vi "Ports Submenu.vi"(11 "menu reference":refnum<k9>) -> ()   [LabVIEW 2017]
panel:
  in  "error in (no error)":errorcluster
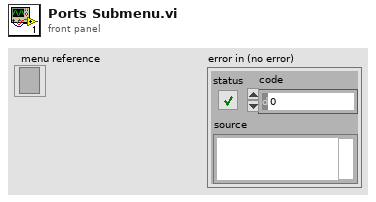
[diagram p1: front panel]
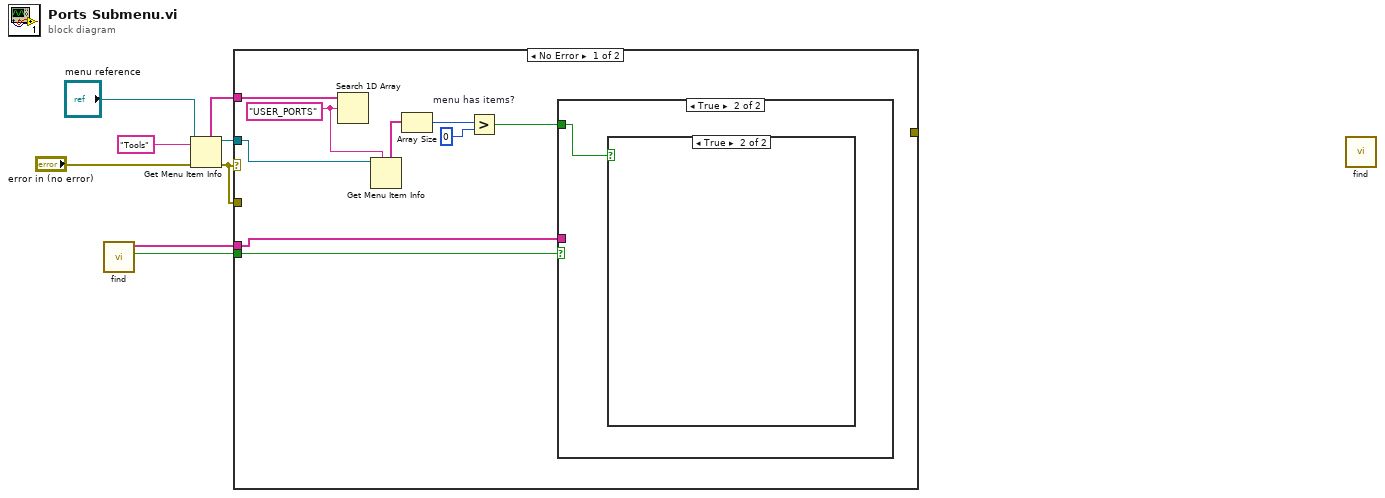
[diagram p0: block diagram]
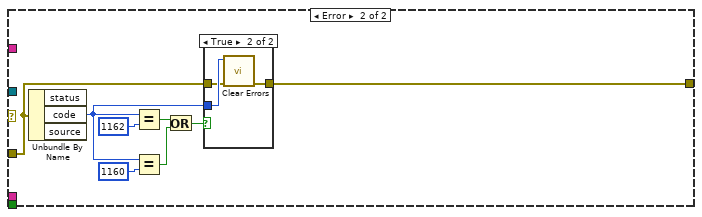
[diagram p5: hidden frame]
diagram:
  n1 = call "find.vi"() -> ("have devices"=w1:bool, "find list"=w2:string[])  [unwired: 9 in, 1 out]
  n2 = Get Menu Item Info(7:"Tools" ("item tag"), 8:"error in (no error)", 11:"menu reference") -> (0:w6:errorcluster, 3:w3:refnum<k9>, 5:w5:string[])  [unwired: 4 out]
  n3 = case shown="No Error" w6 {
    tunnel: w6 -> [_ w21]
    tunnel: [_ w20] -> _
    tunnel: w5 -> [w17 _]
    tunnel: w3 -> [w16 _]
    tunnel: w2 -> [w9 _]
    tunnel: w1 -> [w11 _]
    frame No Error {
      w15 = "USER_PORTS"
      n4 = Search 1D Array(1D array=w17, element=w15) -> ()  [unwired: 1 in, 1 out]
      n5 = Get Menu Item Info(7:w15, 11:w16) -> (5:w14:string[])  [unwired: 1 in, 6 out]
      n6 = Array Size(array=w14) -> (size(s)=w13:i32)
      n7 = Greater? "menu has items?"(x=w13, y=0) -> (0:w10:bool)
      n8 = case shown="True" w11 {
        tunnel: w10 -> [w18 w19]
        tunnel: w9 -> [_ _]
        frame False {
          n9 = case shown="True" w18 {
            frame False {
              # "There are no menu items and no devices. \nSo we do nothing"
            }
            frame True {
              # "There a menu items but no devices. \nSo we remove the menu items."
            }
          }
        }
        frame True {
          n10 = case shown="True" w19 {
            frame False {
            }
            frame True {
            }
          }
        }
      }
    }
    frame Error {
      n11 = Unbundle By Name(w21) -> ("code"=w25:i32)  [unwired: 2 out]
      n12 = Equal?(x=w25, y=1162) -> (x = y?=w23:bool)
      n13 = Equal?(x=w25, y=1160) -> (x = y?=w24:bool)
      n14 = Or(x=w23, y=w24) -> (x .or. y?=w22:bool)
      n15 = case shown="True" w22 {
        tunnel: w25 -> [_ w30]
        tunnel: w21 -> [_ w29]
        tunnel: [_ w28] -> w20
        frame False {
        }
        frame True {
          n16 = call <vilib>:"Clear Errors.vi"("error in (no error)"=w29, "specific error code to clear (0: all)"=w30) -> ("error out"=w28:errorcluster)  [unwired: 4 in, 1 out]
        }
      }
    }
  }
  n17 = call "find.vi"() -> ()  [unwired: 9 in, 3 out]
